vi "simulate_experiment.vi"() -> ()   [LabVIEW 2011]
panel:
  out "output cluster":T1
  in  "frames":i32
  out "average":waveform(dbl)[](graph)
  out "sum":waveform(dbl)[](graph)
  out "mol":waveform(dbl)(graph)
  out "bg":waveform(dbl)(graph)
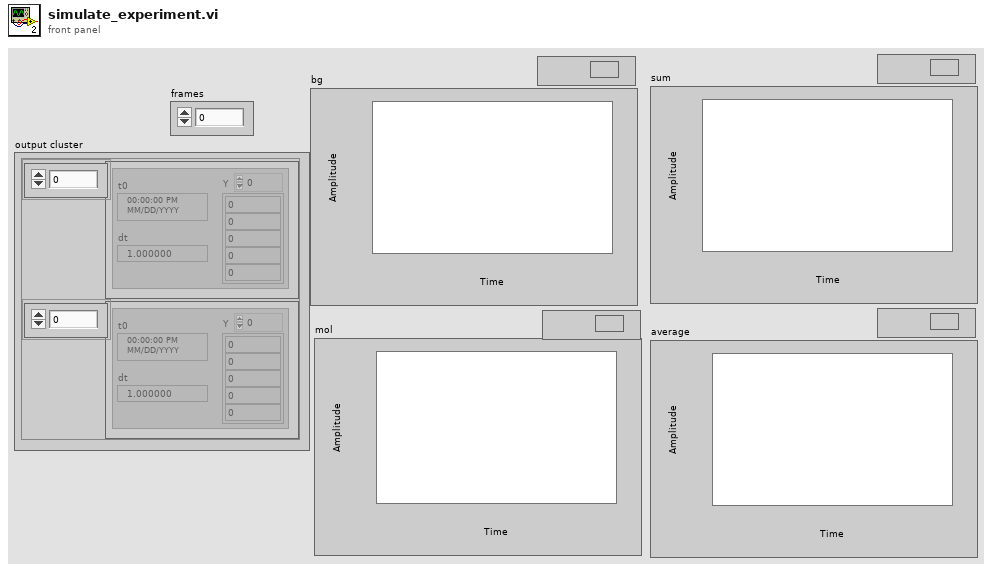
[diagram p1: front panel]
types:
  T1 = cluster{"Array":waveform(dbl)[], "Array":waveform(dbl)[]}
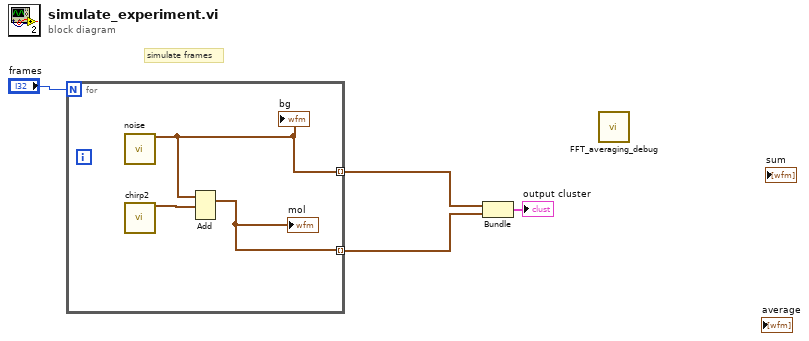
[diagram p0: block diagram]
diagram:
  # "simulate frames"
  n1 = for {
    N: "frames" -> [_]
    tunnel: [w7] -> w1 mode=indexing
    tunnel: [w5] -> w2 mode=indexing
    n2 = call "noise"() -> ("white gaussian noise"=w7:waveform(dbl))  [unwired: 18 in, 1 out]
    "bg" <- w7
    n3 = call "chirp2"() -> ("sine wave"=w6:waveform(dbl))  [unwired: 18 in, 1 out]
    n4 = Add(1:w6, 2:w7) -> (0:w5:waveform(dbl))  [unwired: 1 in, 1 out]
    "mol" <- w5
  }
  n5 = Bundle(w1, w2) -> (→"output cluster":cluster{waveform(dbl)[], waveform(dbl)[]})  [unwired: 1 in]
  n6 = call "FFT_averaging_debug.vi"() -> ()  [unwired: 13 in, 7 out]
